vi "CMI ckd2 Read Error.vi"(8 "error in":errorcluster, 11 "session":T1) -> (0 "error out":errorcluster, 2 "read buffer":string, 3 "session out":T1)   [LabVIEW 2020, in "AWG.lvlib"]
doc: "Tries to read error from instrument error buffer. Generates an error if error found in buffer."
uses:
  AWG.lvlib
  CMI ckd2 Session.ctl
  CMI ckd2 Source Mode.ctl
  <vilib>/Utility/error.llb/Error Cluster From Error Code.vi
  <vilib>/ErrorRing/Error Ring.xnode
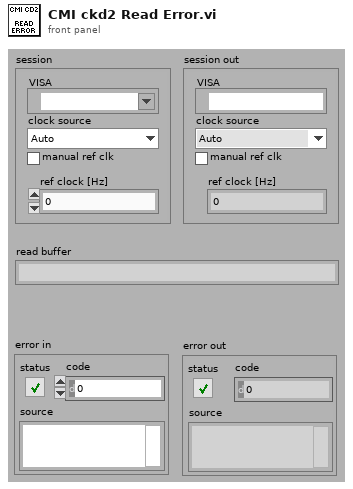
[diagram p1: front panel]
types:
  T1 = typedef "AWG.lvlib/CMI ckd2 Session.ctl" = cluster{"VISA":refnum<visa-resource-name>, "clock source":T2, "manual ref clk":bool, "ref clock [Hz]":dbl}
  T2 = typedef "AWG.lvlib/CMI ckd2 Source Mode.ctl" = enum16{"Auto", "LF clock", "HF clock", "Internal"}
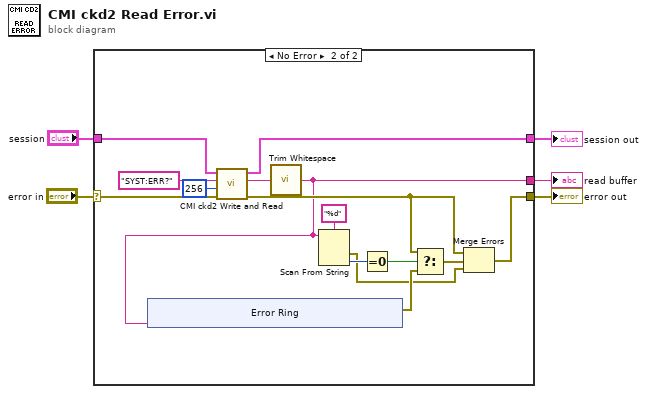
[diagram p0: block diagram]
diagram:
  n1 = case shown="No Error" "error in" {
    selector: "error in" -> [w6 w13]
    tunnel: [w7 w21] -> w2
    tunnel: [w6 w17] -> w5
    tunnel: [_ w9] -> w4
    tunnel: "session" -> [w7 w14]
    frame Error {
    }
    frame No Error {
      n2 = call "CMI ckd2 Write and Read.vi"("error in"=w13, "read byte count (0 - no receive)"=u32 256, "command"="SYST:ERR?" ("write buffer"), "session"=w14) -> ("error out"=w18:errorcluster, "read buffer"=w16:string, "session out"=w21:T1)  [unwired: 5 in]
      n3 = call <vilib>:"Trim Whitespace.vi"("string"=w16) -> ("trimmed string"=w9:string)  [unwired: 1 in]
      n4 = xnode "Error Ring"("parameter 0"=w9) -> ("error out"=w20:errorcluster)
      n5 = Scan From String(format string="%d", input string=w9) -> (error out=w8:errorcluster, output 1=w11:i32)  [unwired: 3 in, 2 out]
      n6 = Equal To 0?(x=w11) -> (x = 0?=w10:bool)
      n7 = Select(t=w18, s=w10, f=w20) -> (s? t:f=w19:errorcluster)
      n8 = Merge Errors(w18, w19, w8) -> (w17:errorcluster)
    }
  }
  "error out" <- w5
  "read buffer" <- w4
  "session out" <- w2
